vi "SendMessageToCaller.vi"(8 "error in (no error)":errorcluster, 11 "TCP_Server_Connection_Handler in":refnum<class "TCP_Server_Connection_Handler.lvclass">) -> (0 "error out":errorcluster, 3 "TCP_Server_Connection_Handler out":refnum<class "TCP_Server_Connection_Handler.lvclass">)   [LabVIEW 2023, in "TCP_Server_Connection_Handler.lvlib" / "TCP_Server_Connection_Handler.lvclass"]
uses:
  TCP_Server_Connection_Handler.lvclass
  TypeDefinitions/ClientMessage.ctl
  TCP_Server_Connection_Handler.lvclass/TCP_Server_Connection_Handler.ctl
  <vilib>/ActorFramework/Actor/Actor.lvclass/Actor.ctl
  TCP_Connections_Controller Messages/MessageRecieved Msg/MessageRecieved Msg.lvclass/MessageRecieved Msg.ctl
  <vilib>/ActorFramework/Message Enqueuer/Message Enqueuer.lvclass/Message Enqueuer.ctl
  <vilib>/ActorFramework/Message Enqueuer/Enqueue.vi
  TCP_Connections_Controller Messages/MessageRecieved Msg/MessageRecieved Msg.lvclass
  <vilib>/ActorFramework/Message Priority Queue/Priority Enqueue.vi
  <vilib>/ActorFramework/Actor/Actor.lvclass
  TCP_Server_Connection_Handler.lvlib
  C:/Program Files (x86)/National Instruments/LabVIEW 2023/vi.lib/ActorFramework/Actor/Actor.lvclass
  C:/Source/LabVIEW/TCP_server/TCP_Server_Connection_Handler/TCP_Server_Connection_Handler/TCP_Server_Connection_Handler.lvclass
  <vilib>/ActorFramework/Stop Msg/Stop Msg.lvclass
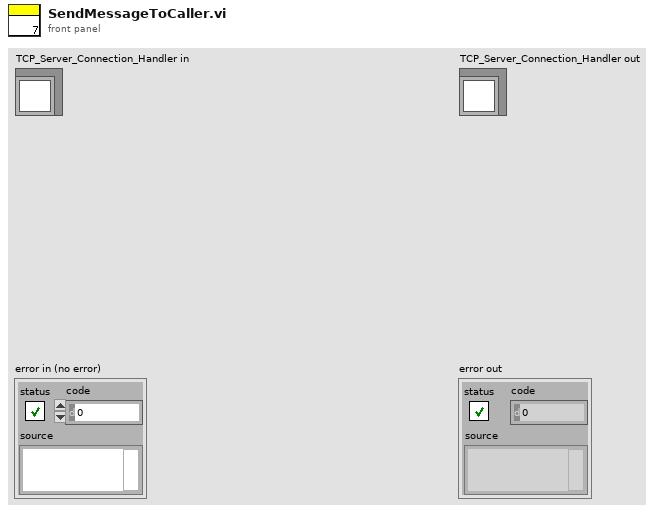
[diagram p1: front panel]
types:
  T1 = typedef "TCP_Server_Connection_Handler.lvlib/ClientMessage.ctl" = cluster{"ConnectionNumber":i32, "ClientIP":string, "Message":string}
  T2 = typedef "TCP_Listener.lvlib/ConnectionInformation.ctl" = cluster{"Connection number":i32, "Remote Address":string, "Remote Port":u16, "Connection ID":refnum<k5>}
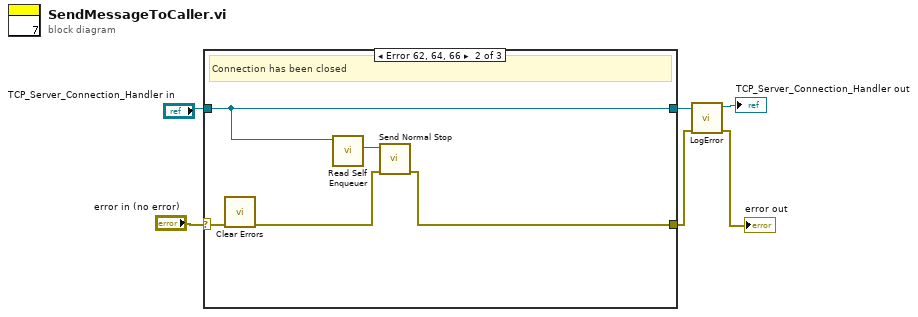
[diagram p0: block diagram]
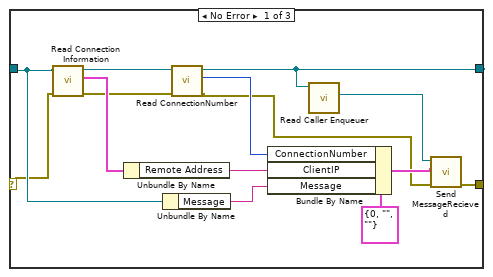
[diagram p2: hidden frame]
diagram:
  n1 = case shown="Error 62, 64, 66" "error in (no error)" {
    selector: "error in (no error)" -> [w9 w23 w27]
    tunnel: [w8 w21 w27] -> w2
    tunnel: [w10 w25 w26] -> w4
    tunnel: "TCP_Server_Connection_Handler in" -> [w11 w25 w26]
    frame No Error {
      n2 = call "Read Connection Information.vi"("error in (no error)"=w9, "TCP_Server_Connection_Handler in"=w11) -> ("error out"=w13:errorcluster, "Connection Information"=w15:T2, "TCP_Server_Connection_Handler out"=w20:refnum<class "TCP_Server_Connection_Handler.lvclass">)  [unwired: 7 in]
      n3 = Unbundle By Name(w15) -> ("Remote Address"=w14:string)
      n4 = Unbundle By Name(w11) -> ("Message"=w7:string)
      n5 = call "Read ConnectionNumber.vi"("error in (no error)"=w13, "TCP_Server_Connection_Handler in"=w20) -> ("error out"=w12:errorcluster, "ConnectionNumber"=w17:i32, "TCP_Server_Connection_Handler out"=w10:refnum<class "TCP_Server_Connection_Handler.lvclass">)  [unwired: 7 in]
      n6 = Bundle By Name(cluster=T1 {"ConnectionNumber"=0, "ClientIP"="", "Message"=""} ("clientMessage"), "ConnectionNumber"=w17, "ClientIP"=w14, "Message"=w7) -> (w16:T1)
      n7 = call <vilib>:"Read Caller Enqueuer.vi"("Actor"=w10) -> ("Caller Enqueuer"=w19:refnum<class "Message Enqueuer.lvclass">)  [unwired: 10 in]
      n8 = call "Send MessageRecieved.vi"("error in (no error)"=w12, "clientMessage"=w16, "Message Enqueuer"=w19) -> ("error out"=w8:errorcluster)  [unwired: 7 in, 1 out]
    }
    frame Error {
      # "Connection has been closed"
      n9 = call <vilib>:"Clear Errors.vi"("error in (no error)"=w23) -> ("error out"=w22:errorcluster)  [unwired: 5 in, 1 out]
      n10 = call <vilib>:"Read Self Enqueuer.vi"("Actor"=w25) -> ("Self Enqueuer"=w24:refnum<class "Message Enqueuer.lvclass">)  [unwired: 10 in]
      n11 = call <vilib>:"Send Normal Stop.vi"("error in (no error)"=w22, "Message Enqueuer"=w24) -> ("error out"=w21:errorcluster)  [unwired: 9 in]
    }
    frame Default {
    }
  }
  n12 = call "LogError.vi"("error in (no error)"=w2, "TCP_Server_Connection_Handler in"=w4) -> ("error out"=→"error out":errorcluster, "TCP_Server_Connection_Handler out"=→"TCP_Server_Connection_Handler out":refnum<class "TCP_Server_Connection_Handler.lvclass">)  [unwired: 8 in]
